vi "LeerBD.vi"(8 "error in (no error)":errorcluster) -> (0 "error out":errorcluster, 2 "BD":T1, 3 "Prueba02 out":refnum<class "Prueba02.lvclass">)   [LabVIEW 2019, in "Prueba02.lvclass"]
uses:
  Prueba02.lvclass
  Controles/BD.ctl
  Base de Datos/SQLiteConnector/SQLiteConnection.lvclass
  Base de Datos/Base de Datos.lvclass
panel:
  in  "Tipo Equipo":enum16{"Sonometro", "Calibrador", "Dosimetro"}(ring)
  out "query":string
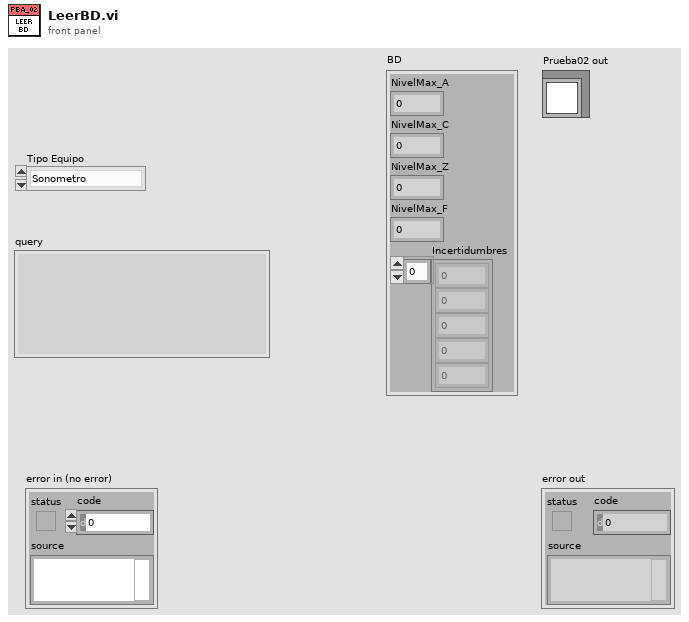
[diagram p1: front panel]
types:
  T1 = typedef "Prueba02.lvclass/BD.ctl" = cluster{"NivelMax_A":dbl, "NivelMax_C":dbl, "NivelMax_Z":dbl, "NivelMax_F":dbl, "Incertidumbres":dbl[]}
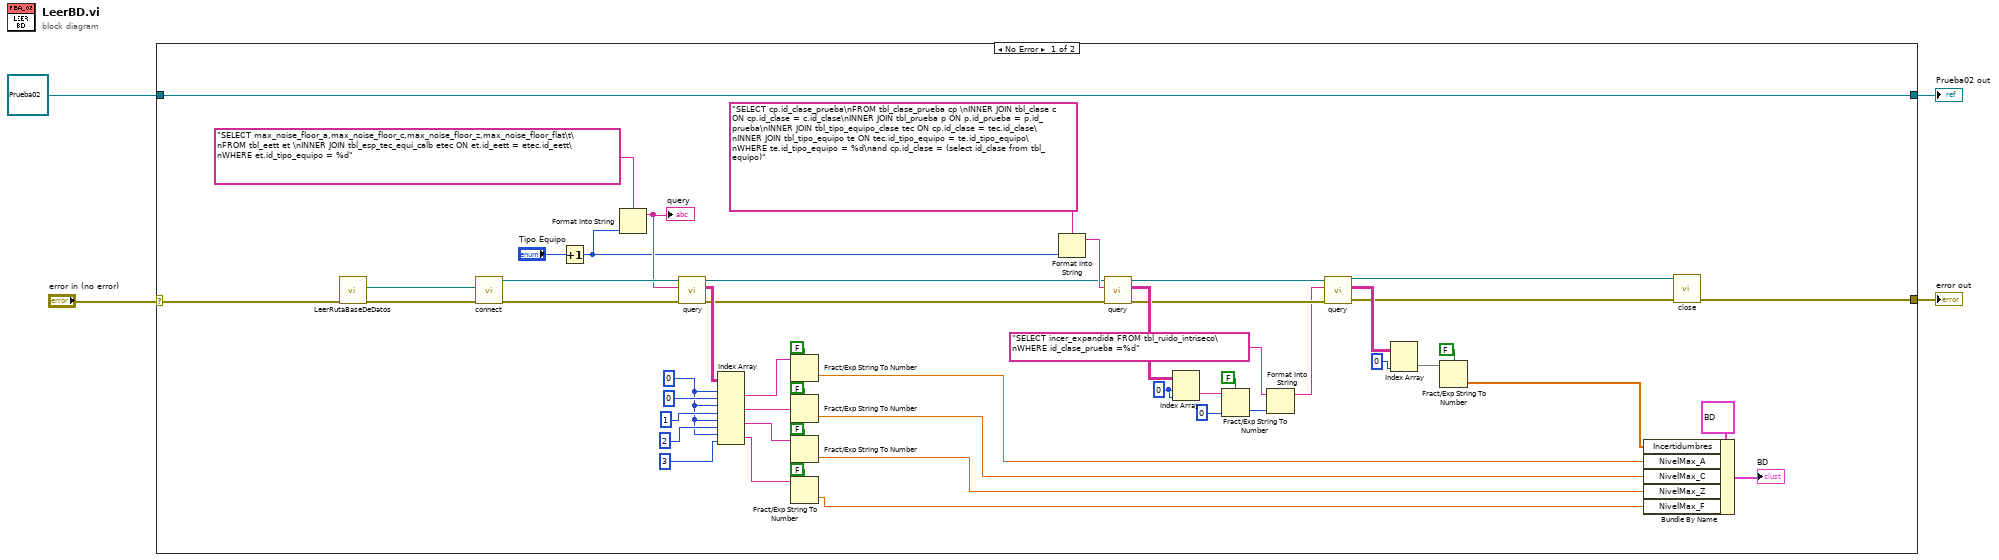
[diagram p0: block diagram]
diagram:
  n1 = case shown="No Error" "error in (no error)" {
    selector: "error in (no error)" -> [w48 w58]
    tunnel: [w17 w58] -> w3
    tunnel: [w56 w57] -> w1
    tunnel: refnum<class "Prueba02.lvclass"> refnum ("Prueba02 in") -> [w56 w57]
    frame No Error {
      w32 = 0 ("index (row)")
      w15 = 0 ("index (row)")
      n2 = call "LeerRutaBaseDeDatos.vi"("error in (no error)"=w48) -> ("error out"=w51:errorcluster, "Database Path"=w50:path)  [unwired: 9 in]
      n3 = call "connect.vi"("error in (no error)"=w51, "Database Path"=w50) -> ("error out"=w53:errorcluster, "object out"=w54:refnum<class "SQLiteConnection.lvclass">)  [unwired: 8 in]
      n4 = Increment(x="Tipo Equipo") -> (x+1=w33:enum16{"Sonometro", "Calibrador", "Dosimetro"})
      n5 = Format Into String(format string="SELECT max_noise_floor_a,max_noise_floor_c,max_noise_floor_z,max_noise_floor_flat\t\nFROM tbl_eett et \nINNER JOIN tbl_esp_tec_equi_calb etec ON et.id_eett = etec.id_eett\nWHERE et.id_tipo_equipo = %d", w33) -> (resulting string=w52:string)  [unwired: 2 in, 1 out]
      "query" <- w52
      n6 = call "query.vi"("error in (no error)"=w53, "SQL Statement"=w52, "object in"=w54) -> ("error out"=w34:errorcluster, "result"=w38:string[][], "object out"=w35:refnum<class "SQLiteConnection.lvclass">)  [unwired: 5 in, 1 out]
      n7 = Index Array(array=w38, index (row) #1=w15, index (col) #1=0 ("disabled index (col)"), index (row) #2=w15, index (col) #2=1 ("disabled index (col)"), index (row) #3=w15, index (col) #3=2 ("index (col)"), index (row) #4=w15, index (col) #4=3 ("index (col)")) -> (element #1=w45:string, element #2=w44:string, element #3=w40:string, element #4=w12:string)
      n8 = Fract/Exp String To Number(use system decimal point (T)=FALSE, string=w45) -> (number=w9:dbl)  [unwired: 2 in, 1 out]
      n9 = Fract/Exp String To Number(use system decimal point (T)=FALSE, string=w44) -> (number=w8:dbl)  [unwired: 2 in, 1 out]
      n10 = Fract/Exp String To Number(use system decimal point (T)=FALSE, string=w40) -> (number=w7:dbl)  [unwired: 2 in, 1 out]
      n11 = Fract/Exp String To Number(use system decimal point (T)=FALSE, string=w12) -> (number=w6:dbl)  [unwired: 2 in, 1 out]
      n12 = Format Into String(format string="SELECT cp.id_clase_prueba\nFROM tbl_clase_prueba cp \nINNER JOIN tbl_clase c ON cp.id_clase = c.id_clase\nINNER JOIN tbl_prueba p ON p.id_prueba = p.id_prueba\nINNER JOIN tbl_tipo_equipo_clase tec ON cp.id_clase = tec.id_clase\nINNER JOIN tbl_tipo_equipo te ON tec.id_tipo_equipo = te.id_tipo_equipo\nWHERE te.id_tipo_equipo = %d\nand cp.id_clase = (select id_clase from tbl_equipo)", w33) -> (resulting string=w36:string)  [unwired: 2 in, 1 out]
      n13 = call "query.vi"("error in (no error)"=w34, "SQL Statement"=w36, "object in"=w35) -> ("error out"=w21:errorcluster, "result"=w26:string[][], "object out"=w22:refnum<class "SQLiteConnection.lvclass">)  [unwired: 5 in, 1 out]
      n14 = Index Array(array=w26, index (row)=w32, index (col)=w32) -> (element=w30:string)
      n15 = Fract/Exp String To Number(use system decimal point (T)=FALSE, string=w30, default (0 dbl)=0 ("index (row)")) -> (number=w29:i32)  [unwired: 1 in, 1 out]
      n16 = Format Into String(format string="SELECT incer_expandida FROM tbl_ruido_intriseco\nWHERE id_clase_prueba =%d", w29) -> (resulting string=w20:string)  [unwired: 2 in, 1 out]
      n17 = call "query.vi"("error in (no error)"=w21, "SQL Statement"=w20, "object in"=w22) -> ("error out"=w18:errorcluster, "result"=w23:string[][], "object out"=w19:refnum<class "SQLiteConnection.lvclass">)  [unwired: 5 in, 1 out]
      n18 = Index Array(array=w23, index (col)=0 ("index (row)")) -> (element=w25:string[])  [unwired: 1 in]
      n19 = Fract/Exp String To Number(use system decimal point (T)=FALSE, string=w25) -> (number=w10:dbl[])  [unwired: 2 in, 1 out]
      n20 = Bundle By Name(cluster=T1 {"NivelMax_A"=98.0, "NivelMax_C"=97.0, "NivelMax_Z"=96.0, "NivelMax_F"=99.0, "Incertidumbres"=[1.0, 1.0, 1.0, 1.0]} ("BD"), "Incertidumbres"=w10, "NivelMax_A"=w9, "NivelMax_C"=w8, "NivelMax_Z"=w7, "NivelMax_F"=w6) -> (→"BD":T1)
      n21 = call-dynamic "close.vi"("error in (no error)"=w18, "object in"=w19) -> ("error out"=w17:errorcluster)  [unwired: 8 in, 1 out]
    }
    frame Error {
    }
  }
  "error out" <- w3
  "Prueba02 out" <- w1
